vi "CompressorOutput.vi"   [LabVIEW 2019]
uses:
  47a2bda7-ce34-456f-9ccf-c1151ea95870.vi
  refnums.vi
  GRNF_Compressor.vi
  outputs.vi
  dsdata.vi
types:
  T1 = typedef "WPI_CompressorDevRef.ctl" = cluster{"DevStatus":errorcluster, "Pneumatics Control Module":u8}
  T2 = typedef "WPI_DriverStationRobotMode2.ctl" = enum16{"Autonomous Disabled", "Autonomous Enabled", "Teleop Disabled", "Teleop Enabled", "Disconnected", "Finish", "Test Disabled", "Test Enabled", "Emergency Stopped"}
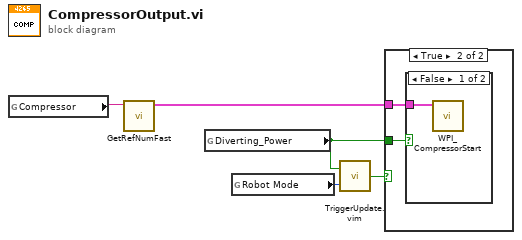
[diagram p0: block diagram]
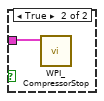
[diagram p3: hidden frame]
diagram:
  n1 = global read "refnums.vi" "Compressor"() -> (w1:string)
  n2 = call-poly "GetRefNumFast.vi"("RefNum Name"=w1) -> ("Device Reference"=w2:T1)  [unwired: 5 in, 1 out]
  n3 = global read "outputs.vi" "Diverting_Power"() -> (w5:bool)
  n4 = global read "dsdata.vi" "Robot Mode"() -> (w3:T2)
  n5 = call "TriggerUpdate.vim"("Robot Mode"=w3, "Trigger"=w5) -> ("Update"=w4:bool)
  n6 = case shown="True" w4 {
    tunnel: w5 -> [_ w7]
    tunnel: w2 -> [_ w6]
    frame False {
    }
    frame True {
      n7 = case shown="False" w7 {
        tunnel: w6 -> [w8 w9]
        frame False {
          n8 = call <vilib>:"WPI_CompressorStart.vi"("CompressorDevRef"=w8) -> ()  [unwired: 9 in, 2 out]
        }
        frame True {
          n9 = call <vilib>:"WPI_CompressorStop.vi"("CompressorDevRef"=w9) -> ()  [unwired: 9 in, 2 out]
        }
      }
    }
  }
